vi "Poll Epics Array.vi"(7 "Message name":string, 8 "error in (no error)":errorcluster, 9 "Shared variable":bool[](array[boolean]), 10 "Epics variable":bool[](array[boolean]), 11 "Queue in":refnum<queue>) -> (0 "error out":errorcluster, 2 "Update?":bool, 3 "Epics variable out":bool[](array[boolean]))   [LabVIEW 2014]
uses:
  Message Queue/Message Cluster.ctl
  Message Queue/Message Queue.lvlib
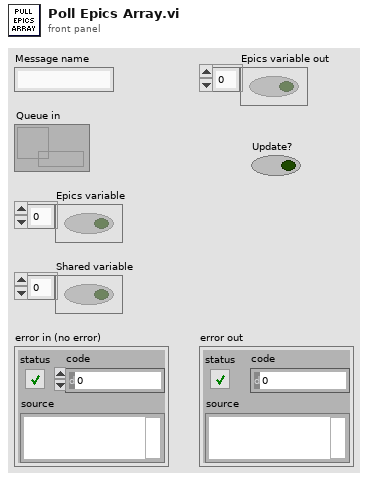
[diagram p1: front panel]
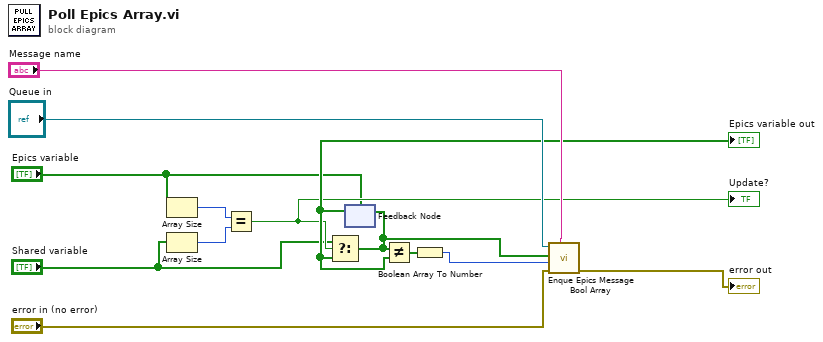
[diagram p0: block diagram]
diagram:
  n1 = Array Size(array="Epics variable") -> (size(s)=w3:i32)
  n2 = Array Size(array="Shared variable") -> (size(s)=w4:i32)
  n3 = Equal?(x=w3, y=w4) -> (x = y?=w9:bool)
  "Update?" <- w9
  n4 = feedback #1("Epics variable") -> (w11:bool[])
  "Epics variable out" <- w11
  n5 = Select(t="Shared variable", s=w9, f=w11) -> (s? t:f=w10:bool[])
  n6 = feedback-in #1(w10) -> ()
  n7 = Not Equal?(x=w10, y=w11) -> (x != y?=w5:bool[])
  n8 = Boolean Array To Number(Boolean array=w5) -> (number=w6:u32)
  n9 = call "Enque Epics Message Bool Array.vi"("Message name"="Message name", "error in (no error)"="error in (no error)", "Numeric"=w6, "Epics variable"=w10, "Queue in"="Queue in") -> ("error out"=→"error out":errorcluster)  [unwired: 6 in]
